vi "Generate XML String for EMV Test.vi"() -> ()   [LabVIEW 2013]
doc: "This example illustrates how to create an XML document and save it as an XML file."
uses:
  <resource>/objmgr/DOMUserDefRef.rc
  <vilib>/xml/NI_XML.lvlib
  <vilib>/xml/Close Reference(Node).vi
  OOP/Report.lvclass
  Hauptprojekt/EMV/controls/Data.ctl
panel:
  in  "time":string
  in  "pruefer":string
  in  "obrn":string
  in  "label":string
  in  "imgPath":string
  in  "Baugruppenname":string
  in  "SegName":string
  in  "Comment":string
  in  "TestName":string
  out "Generated XML":string
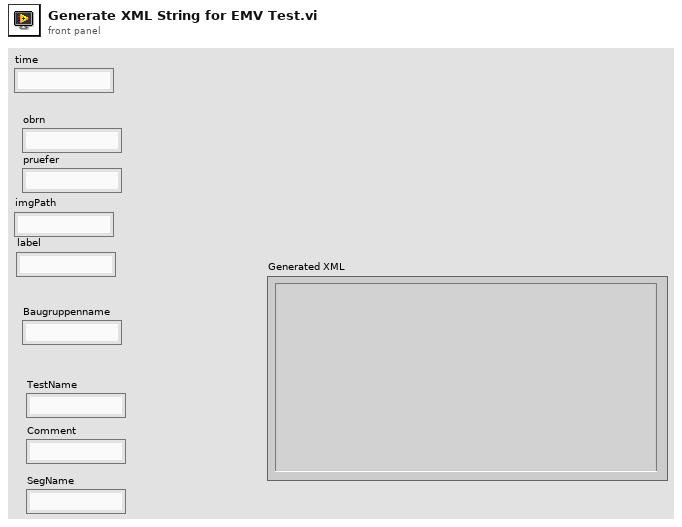
[diagram p1: front panel]
types:
  T1 = typedef "Data.ctl" = cluster{"Report.lvclass":refnum<class "Report.lvclass">, "Test":string, "images":dbl}
  T2 = enum16{"open", "replace", "create", "open or create", "replace or create", "replace or create with confirmation"}
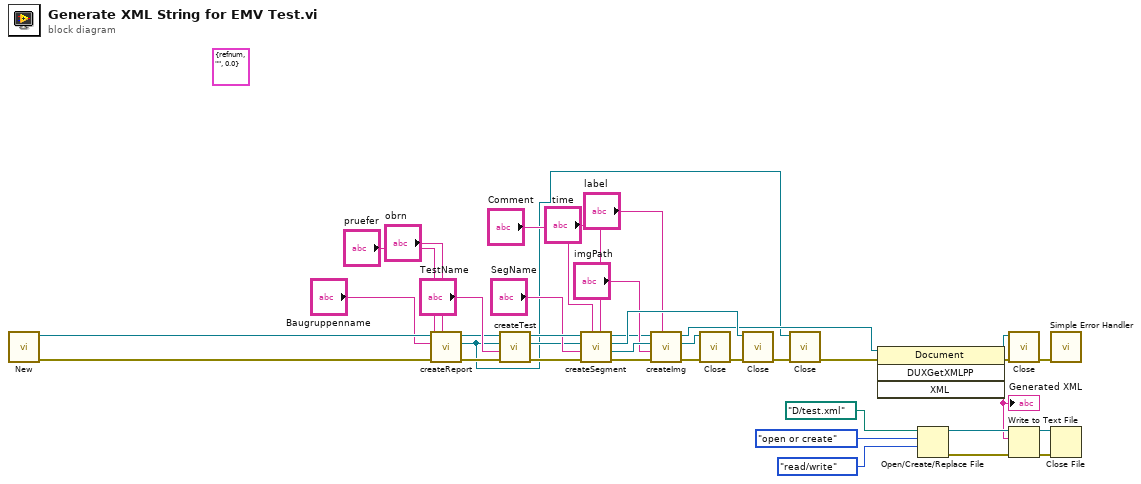
[diagram p0: block diagram]
diagram:
  (unwired) T1 {"Report.lvclass"=refnum, "Test"="", "images"=0.0} ("Data")
  n1 = call <vilib>:"New.vi"() -> ("error out"=w20:errorcluster, "DOM document out"=w19:refnum<k20>)  [unwired: 1 in, 7 out]
  n2 = call "createReport.vi"("obrn"="obrn", "error in (no error)"=w20, "pruefer"="pruefer", "Baugruppenname"="Baugruppenname", "DOM Document"=w19) -> ("error out"=w17:errorcluster, "Report ref"=w2:refnum<k20>, "dup DOM Document"=w18:refnum<k20>)  [unwired: 4 in]
  n3 = call "createTest.vi"("error in (no error)"=w17, "TestName"="TestName", "report ref"=w2, "DOM document"=w18) -> ("error out"=w32:errorcluster, "test ref"=w3:refnum<k20>, "dup DOM document"=w33:refnum<k20>)  [unwired: 4 in, 1 out]
  n4 = call "createSegment.vi"("time"="time", "Comment"="Comment", "error in (no error)"=w32, "SegName"="SegName", "test ref"=w3, "DOM document"=w33) -> ("error out"=w15:errorcluster, "seg ref"=w14:refnum<k20>, "dup test ref"=w31:refnum<k20>, "dup DOM document"=w11:refnum<k20>)  [unwired: 2 in]
  n5 = call "createImg.vi"("label"="label", "error in (no error)"=w15, "link"="imgPath", "seg ref"=w14, "DOM document"=w11) -> ("error out"=w9:errorcluster, "dup seg ref"=w8:refnum<k20>, "dup DOM document"=w4:refnum<k20>)  [unwired: 4 in]
  n6 = call-poly <vilib>:"Close.vi"("error in (no error)"=w9, "node"=w8) -> ("error out"=w10:errorcluster)  [unwired: 7 out]
  n7 = call-poly <vilib>:"Close.vi"("error in (no error)"=w10, "node"=w31) -> ("error out"=w35:errorcluster)  [unwired: 7 out]
  n8 = call-poly <vilib>:"Close.vi"("error in (no error)"=w35, "node"=w2) -> ("error out"=w1:errorcluster)  [unwired: 7 out]
  n9 = invoke class="Document" method="DUXGetXMLPP"(reference=w4, error in=w1) -> (reference out=w37:refnum<k20>, error out=w38:errorcluster, "XML"=w21:string)  [unwired: 2 in, 1 out]
  "Generated XML" <- w21
  n10 = Open/Create/Replace File(file path (use dialog)=path "D:/test.xml" ("Dateipfad (Dialog verwenden)"), operation (0:open)=T2."open or create" ("Operation (0:Öffnen)"), access (0:read/write)=enum16{"read/write", "read-only", "write-only"}."read/write" ("Zugriff (0:Lesen/Schreiben)")) -> (refnum out=w23:refnum<file>, error out=w24:errorcluster)  [unwired: 3 in, 1 out]
  n11 = call-poly <vilib>:"Close.vi"("error in (no error)"=w38, "node"=w37) -> ("error out"=w36:errorcluster)  [unwired: 7 out]
  n12 = Write to Text File(file (use dialog)=w23, text=w21, error in=w24) -> (refnum out=w28:refnum<file>, error out=w27:errorcluster)  [unwired: 1 in, 1 out]
  n13 = call <vilib>:"Simple Error Handler.vi"("error in (no error)"=w36) -> ()  [unwired: 1 in, 8 out]
  n14 = Close File(refnum=w28, error in=w27) -> ()  [unwired: 2 out]
